vi "sum.vi"() -> ()   [LabVIEW 2017]
panel:
  out "sum":i32
  in  "N":i32
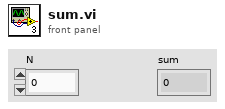
[diagram p1: front panel]
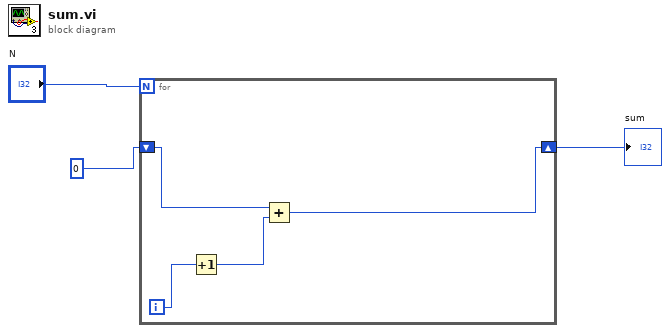
[diagram p0: block diagram]
diagram:
  n1 = for {
    N: "N" -> [_]
    shift-right: [w4] -> w2
    shift-left: 0 -> [w5]
    i -> [w7]
    n2 = Increment(x=w7) -> (x+1=w6:i32)
    n3 = Add(x=w5, y=w6) -> (x+y=w4:i32)
  }
  "sum" <- w2
